vi "Calc Eval.vi"(8 "error in (no error)":errorcluster, 10 "Inputs":dbl[](array[numeric]), 11 "Max Calc in":refnum<class "Max Calc.lvclass">) -> (0 "error out":errorcluster, 1 "Additional Updates":T1[](array[typedef]), 2 "Result":dbl, 3 "Max Calc out":refnum<class "Max Calc.lvclass">)   [LabVIEW 2020, in "VolatusCalcs.lvlib" / "Max Calc.lvclass"]
uses:
  Max Calc.lvclass
  Max Calc.lvclass/Max Calc.ctl
  Calculation/Additional Update.ctl
  Calculation/Calculation.lvclass
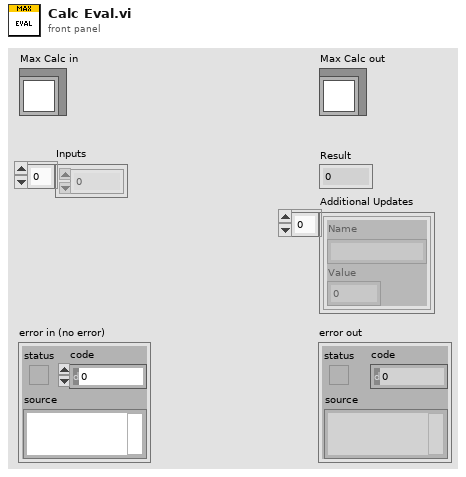
[diagram p1: front panel]
types:
  T1 = typedef "VolatusCalcs.lvlib/Calculation.lvclass/Additional Update.ctl" = cluster{"Name":string, "Value":dbl}
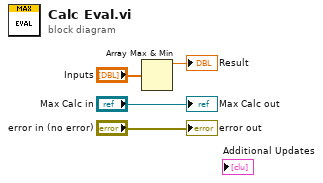
[diagram p0: block diagram]
diagram:
  n1 = Array Max & Min(array="Inputs") -> (max value=→"Result":dbl)  [unwired: 3 out]
  "error out" <- "error in (no error)"
  "Max Calc out" <- "Max Calc in"
